vi "test Search 2D Array for Element.vi"(8 "error in (no error)":errorcluster, 11 "TestCase in":refnum<class "Utility VIs tests.lvclass">) -> (0 "error out":errorcluster, 3 "TestCase out":refnum<class "Utility VIs tests.lvclass">)   [LabVIEW 2014, in "Utility VIs tests.lvclass"]
uses:
  Utility VIs tests.lvclass
  <vilib>/addons/_JKI Toolkits/VI Tester/TestCase.llb/TestCase.lvclass
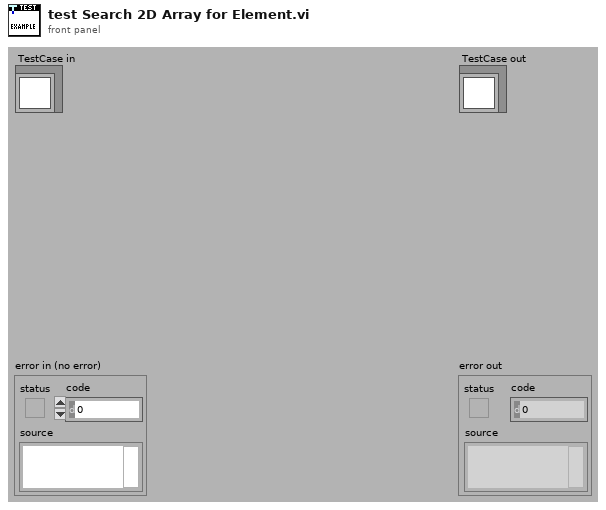
[diagram p1: front panel]
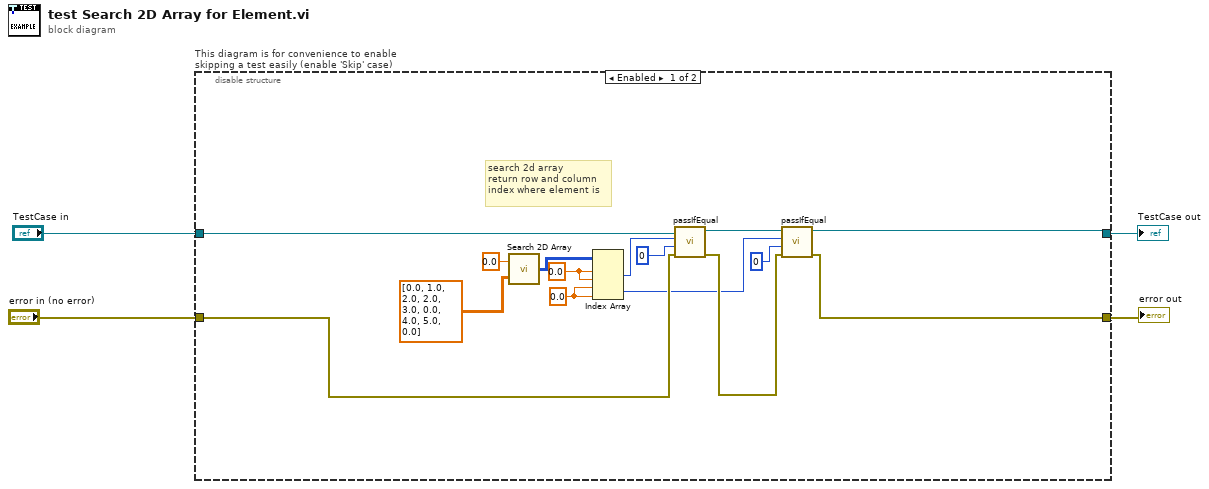
[diagram p0: block diagram]
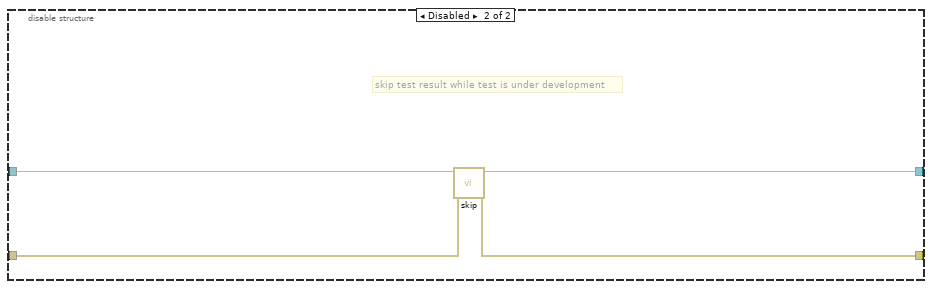
[diagram p2: hidden frame]
diagram:
  n1 = disable-structure "This diagram is for convenience to enable skipping a test easily (enable 'Skip' case)" shown="Enabled" {
    disable-tunnel: "TestCase in" -> [w17 w23]
    disable-tunnel: [w12 w21] -> w1
    disable-tunnel: [w13 w22] -> w3
    disable-tunnel: "error in (no error)" -> [w15 w20]
    frame Enabled {
      w9 = 0.0 ("Element")
      w10 = 0.0 ("Element")
      # "search 2d array\nreturn row and column\nindex where element is"
      n2 = call "Search 2D Array.vi"("Array"=dbl[][] [[0.0, 1.0, 2.0], [2.0, 3.0, 0.0], [4.0, 5.0, 0.0]], "Element"=0.0) -> ("Locations"=w11:i32[][])
      n3 = Index Array(array=w11, index (row) #1=w10, index (col) #1=w10, index (row) #2=w9, index (col) #2=w9) -> (element #1=w8:i32, element #2=w6:i32)
      n4 = call-dynamic "passIfEqual.vi"("error in (no error)"=w15, "y"=0 ("Element"), "x"=w8, "TestCase in"=w17) -> ("error out"=w14:errorcluster, "TestCase out"=w16:refnum<class "Utility VIs tests.lvclass">)  [unwired: 6 in]
      n5 = call-dynamic "passIfEqual.vi"("error in (no error)"=w14, "y"=0 ("Element"), "x"=w6, "TestCase in"=w16) -> ("error out"=w13:errorcluster, "TestCase out"=w12:refnum<class "Utility VIs tests.lvclass">)  [unwired: 6 in]
    }
    frame Disabled {
      # "skip test result while test is under development"
      n6 = call <vilib>:"skip.vi"("error in (no error)"=w20, "TestCase in"=w23) -> ("error out"=w22:errorcluster, "TestCase out"=w21:refnum<class "Utility VIs tests.lvclass">)  [unwired: 8 in]
    }
  }
  "error out" <- w3
  "TestCase out" <- w1
